vi "Get_RegData_Value.vi"(8 "error in (no error)":errorcluster, 11 "RegData_I32 in":refnum<class "IB_RegData_I32.lvclass">) -> (0 "error out":errorcluster, 1 "type":string, 2 "Val":string, 3 "RegData_I32 out":refnum<class "IB_RegData_I32.lvclass">)   [LabVIEW 2020, in "IB_RegData_I32.lvclass"]
uses:
  <vilib>/AppBuilder/IB_Classes/RegData/RegData_I32/IB_RegData_I32.lvclass
  <vilib>/AppBuilder/IB_Classes/RegData/RegData_I32/IB_RegData_I32.lvclass/IB_RegData_I32.ctl
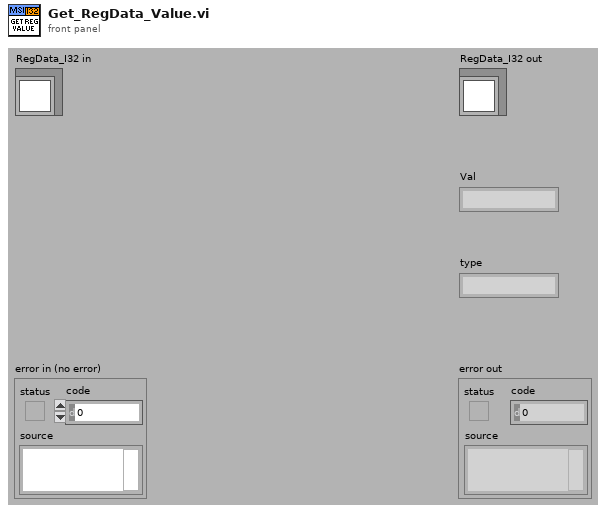
[diagram p1: front panel]
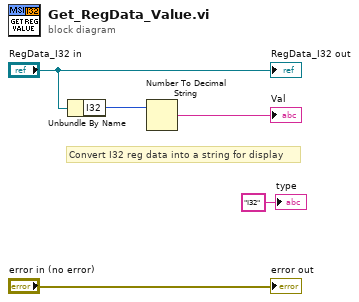
[diagram p0: block diagram]
diagram:
  # "Convert I32 reg data into a string for display"
  n1 = Unbundle By Name("RegData_I32 in") -> ("I32"=w3:i32)
  n2 = Number To Decimal String(number=w3) -> (decimal integer string=→"Val":string)  [unwired: 1 out]
  "error out" <- "error in (no error)"
  "RegData_I32 out" <- "RegData_I32 in"
  "type" <- "I32" ("type")
